vi "Close.vi"(8 "error in (no error)":errorcluster, 11 "NI Digital in":refnum<class "NI Analog Out.lvclass">) -> (0 "error out":errorcluster, 3 "NI Digital out":refnum<class "NI Analog Out.lvclass">)   [LabVIEW 2018, in "NI Analog Out.lvclass"]
doc: "NI Analog Out.lvclass:Close.vi\n\nThis is the Close VI for the NI Analog Out class.\n\nInstrument Communication Module Version 1.0\nOctober, 2020 Original Code Consulting Davita Bird\n www.originalcode.com"
uses:
  NI Analog Out.lvclass
  NI Analog Out.lvclass/NI Analog Out.ctl
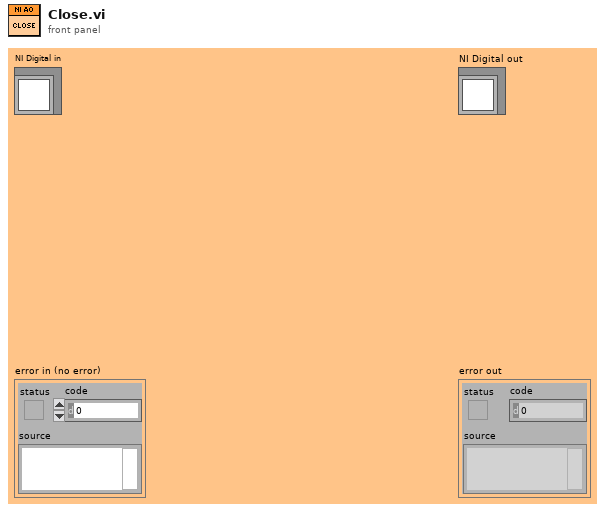
[diagram p1: front panel]
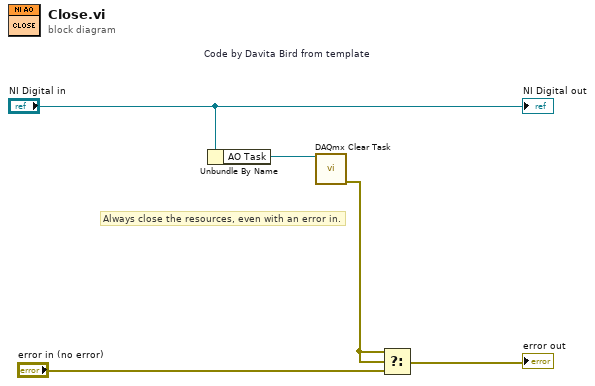
[diagram p0: block diagram]
diagram:
  # "Always close the resources, even with an error in."
  n1 = Unbundle By Name "Code by Davita Bird from template"("NI Digital in") -> ("AO Task"=w4:refnum<k21>)
  n2 = call <vilib>:"DAQmx Clear Task.vi"("task in"=w4) -> ("error out"=w3:errorcluster)  [unwired: 14 in]
  n3 = Select(t=w3, s=w3, f="error in (no error)") -> (s? t:f=→"error out":errorcluster)
  "NI Digital out" <- "NI Digital in"
